vi "RampSlow.vi"() -> ()   [LabVIEW 2016]
uses:
  controls/Enum.ctl
  <vilib>/rvi/errors/niLvFpgaAdjustHostInterfaceError.vi
  <vilib>/rvi/interface/nirviReadWriteControl/nirviReadWriteControl.xnode
  controls/FPGAVIreferenceTypeDef.ctl
  FPGA Bitfiles/qnmController797_usbRIO_controllerFPGAmu-19072018.lvbitx
  Course Project/support/Message Queue/Message Queue.lvlib
  controllerFPGA_multiTarget.vi
  <vilib>/rvi/interface/nirviCloseFPGA/nirviCloseFPGA.xnode
  NiFpgaLv.dll
  <vilib>/rvi/interface/nirviMethod/nirviMethod.xnode
  <vilib>/FPGAPlugInAG/USB-7856R OEM/niLvFpga_AcknowledgeIrq_USB-7856R OEM.vi
  <vilib>/rvi/interface/nirviMethod/StockFPGA_InlinedMethodWaitForSingleIRQ.vi
  <vilib>/FPGAPlugInAG/USB-7856R OEM/niLvFpga_WaitOnIrq_USB-7856R OEM.vi
  <vilib>/FPGAPlugInAG/USB-7856R OEM/niLvFpga_Close_USB-7856R OEM.vi
panel:
  in  "SecureTip":T1 {"Sign" items=[">", "<"]; "Secure tip signal" items=["Vert. Deflection (V)", "Horiz. Deflection (V)", "Input 1", "Input 2"]; "Max-min-Tip" format="%#.2p"}
  in  "Curves 2":i32(listbox)
  in  "Spectroscopy":enum32{"Spectroscopy"}(tab)
  in  "Fwd sweep":bool=TRUE
  in  "Parameters":T2={"Start"=-1e-06, "Distance"=2e-07, "Points"=256.0, "Fwd"=0.0, "Bwd"=0.0, "Pause"=0.0} {"Pause" format="%.0ps"; "Bwd" format="%.0pm/s"; "Distance" format="%#.3pm"; "Start" format="%#.3pm"; "Fwd" format="%.0pm/s"}
  in  "ChannelDisplay2":u16(ring)=1 items=["AI0", "AI1", "AI3", "AI2"]
  in  "ChannelDisplay":u16(ring) items=["AI0", "AI1", "AI3", "AI2"]
  in  "Dec":dbl=1.0 format="%.0p"
  out "ForceCurves 2":cluster{dbl[], dbl[]}[](graph)
  out "ForceCurves":cluster{dbl[], dbl[]}[](graph)
  out "Ramping?":bool
  in  "Bwd sweep":bool=TRUE
  in  "Output":enum16{"Z", "Bias", "..."}(ring)
  in  "Channels":i32[](listbox)=[0, 1, 2, 3]
  in  "Actions":T3={"Play"=FALSE, "Stop"=FALSE, "Loop"=FALSE, "Sweeps"=1.0} {"Sweeps" min=1.0 format="%#.0f"}
  in  "Saving":T4={"#"=0, "Name"="", "Path"=path "C:/ForceCurves", "Autosave"=FALSE, "Save"=FALSE} {"#" format="%03.0f"}
  in  "Curves":T5={"Plot1"={"Apply"=FALSE, "Delete"=FALSE, "Show"=TRUE}, "Plot2"={"Apply"=FALSE, "Delete"=FALSE, "Show"=TRUE}}
  in  "CalculateSlope":bool
  out "1/Slope":dbl format="%#_5pm/V"
  out "B":cluster{"Y":dbl, "X":dbl} {"X" format="%#_2p"; "Y" format="%#_2p"}
  out "A":cluster{"Y":dbl, "X":dbl} {"X" format="%#_2p"; "Y" format="%#_2p"}
  # "Secure tip"
  # "Spectroscopy"
  # "Ramp"
  # "Saving"
  # "Cursors"
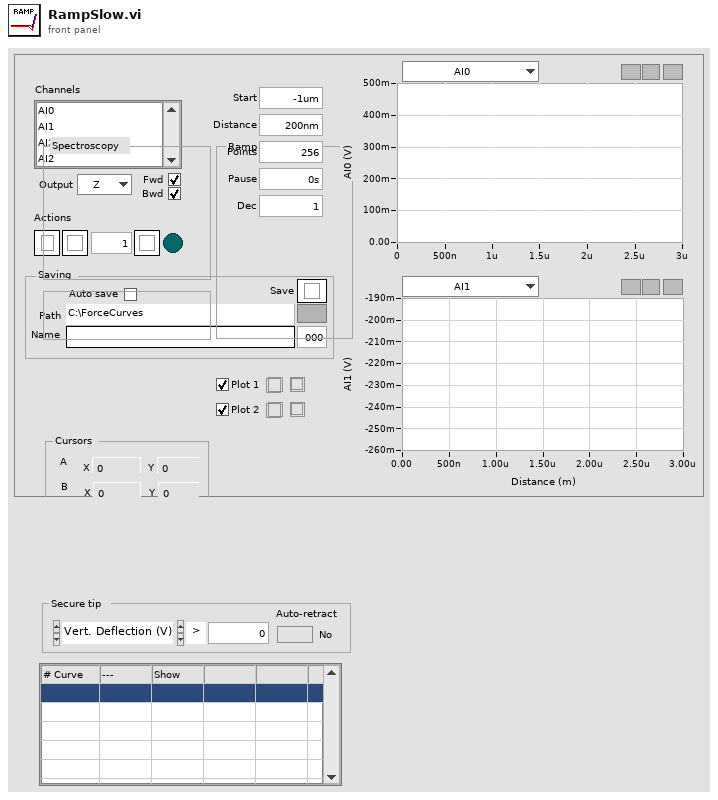
[diagram p1: front panel]
types:
  T1 = cluster{"Max-min-Tip":dbl, "Secure tip signal":u16, "Sign":u16, "Auto-retract":bool}
  T2 = cluster{"Start":dbl, "Distance":dbl, "Points":dbl, "Fwd":dbl, "Bwd":dbl, "Pause":dbl}
  T3 = cluster{"Play":bool, "Stop":bool, "Loop":bool, "Sweeps":dbl}
  T4 = cluster{"#":i64, "Name":string, "Path":path, "Autosave":bool, "Save":bool}
  T5 = cluster{"Plot1":cluster{"Apply":bool, "Delete":bool, "Show":bool}, "Plot2":cluster{"Apply":bool, "Delete":bool, "Show":bool}}
  T6 = typedef "Message Queue.lvlib/All Message Queues.ctl" = cluster{"IU":refnum<queue>}
  T7 = typedef "LVPointDoubleTypeDef.ctl" = cluster{"Cursor X":dbl, "Cursor Y":dbl}
  T8 = typedef "Enum.ctl" = enum16{"Init", "Read", "Write"}
  T9 = enum8{"Enabled", "Disabled", "Disabled and Grayed Out"}
  T10 = enum16{"open", "replace", "create", "open or create", "replace or create", "replace or create with confirmation"}
  T11 = cluster{"calibName":string[], "calibParameters":cluster{"Sensitivity":cluster{"Sens X":dbl, "Sens Y":dbl, "Sens Z":dbl}, "Range":cluster{"Range X":dbl, "Range Y":dbl, "Range Z":dbl}, "HV gain":cluster{"HV gain X":dbl, "HV gain Y":dbl, "HV gain Z":dbl}}[], "calibIndex":i32}
  T12 = cluster{"Sensitivity":cluster{"Sens X":dbl, "Sens Y":dbl, "Sens Z":dbl}, "Range":cluster{"Range X":dbl, "Range Y":dbl, "Range Z":dbl}, "HV gain":cluster{"HV gain X":dbl, "HV gain Y":dbl, "HV gain Z":dbl}}[]
  T13 = cluster{"Sensitivity":cluster{"Sens X":dbl, "Sens Y":dbl, "Sens Z":dbl}, "Range":cluster{"Range X":dbl, "Range Y":dbl, "Range Z":dbl}, "HV gain":cluster{"HV gain X":dbl, "HV gain Y":dbl, "HV gain Z":dbl}}
  T14 = typedef "FPGAVIreferenceTypeDef.ctl" = refnum<k20>
  T15 = cluster{"enableManualMotion":bool, "doMove":bool, "integratorTarget":fxp<+/-,22,2>, "clocks":cluster{"inverseDecimation":fxp<+,22,0>, "decimation":u16, "waveSize":u16, "pixelDecimation":u16}}
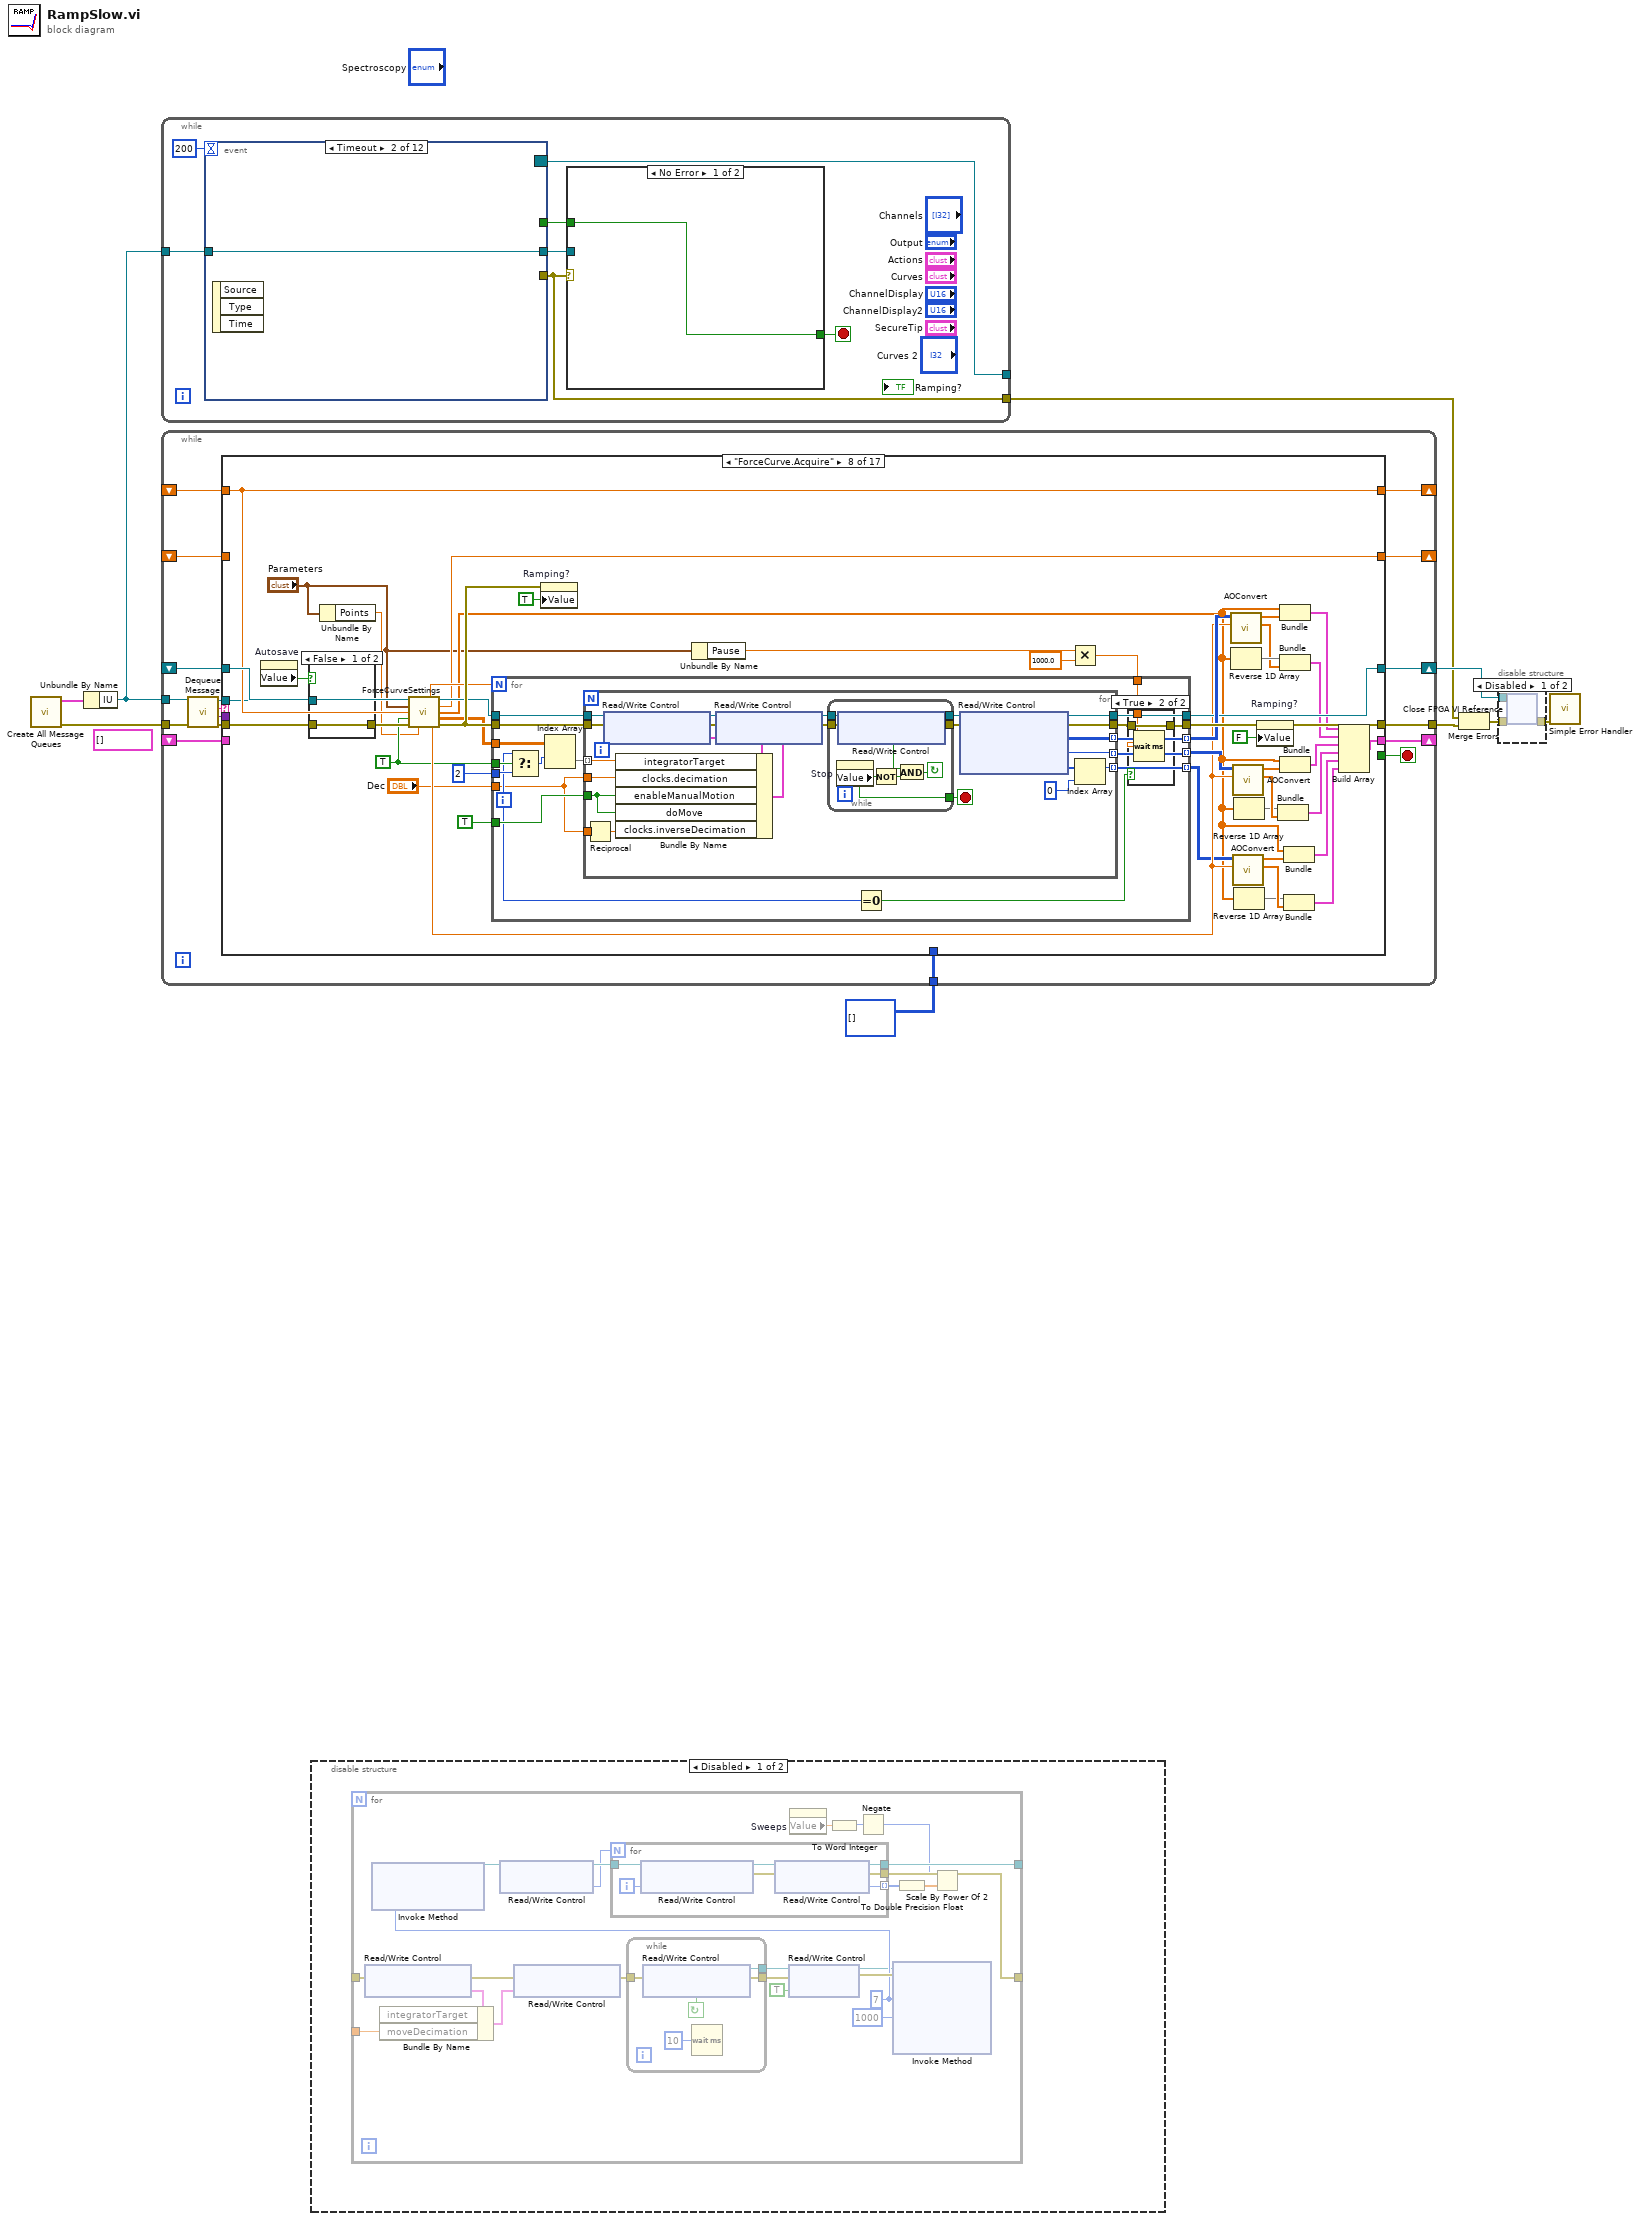
[diagram p0: block diagram]
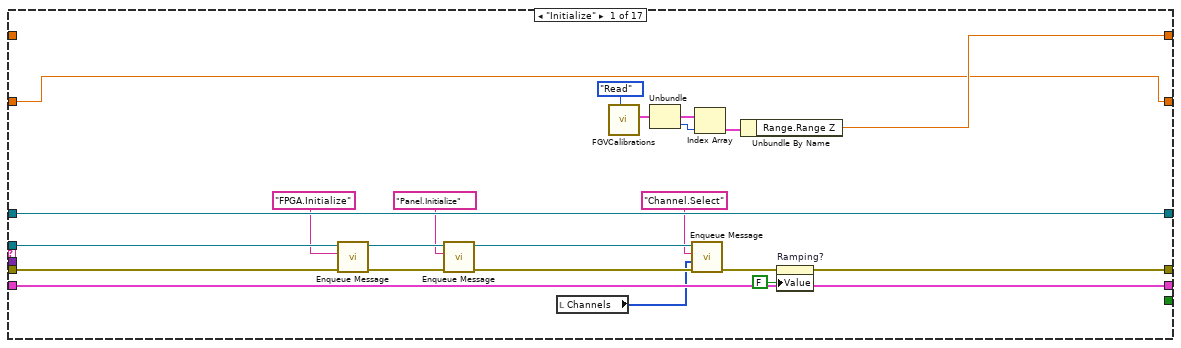
[diagram p4: hidden frame]
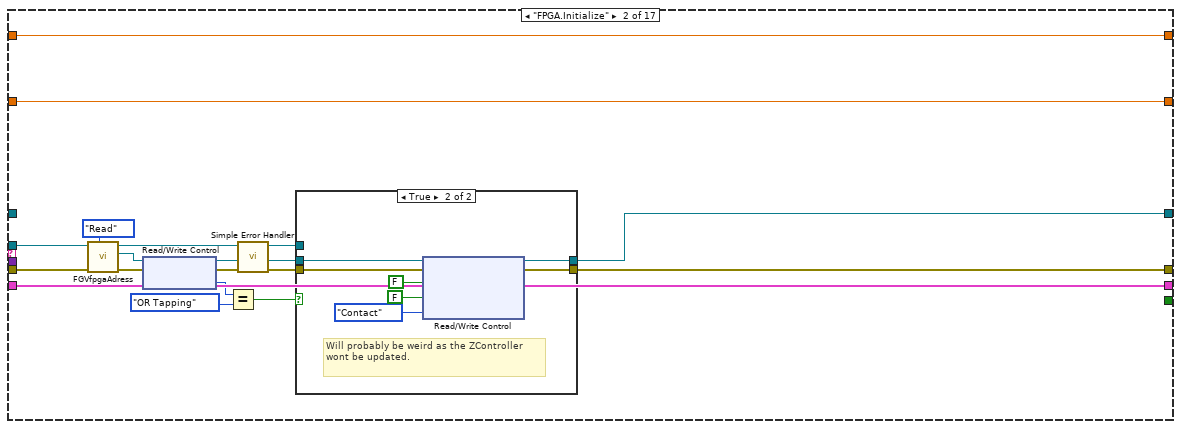
[diagram p5: hidden frame]
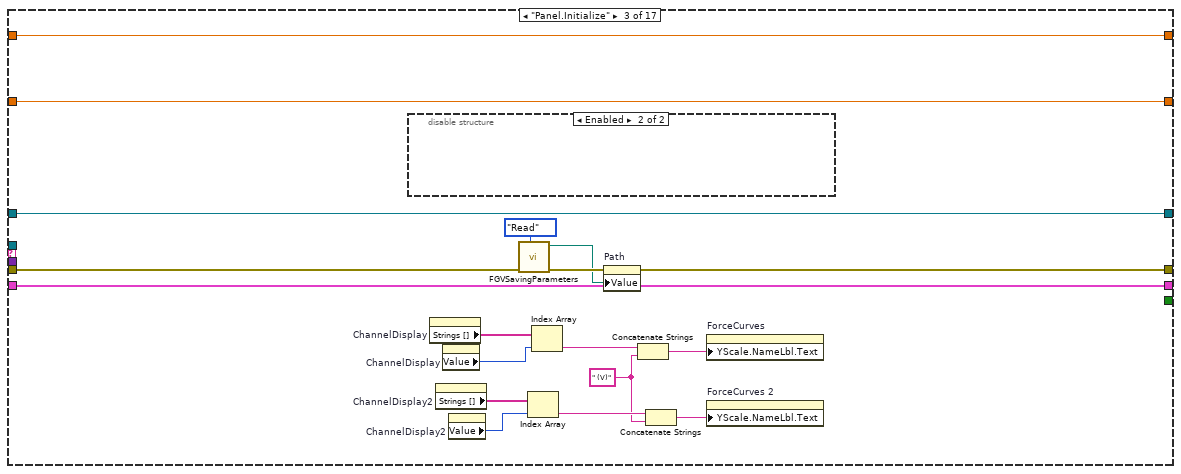
[diagram p7: hidden frame]
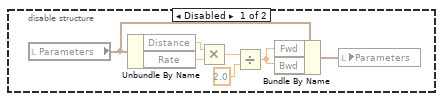
[diagram p8: hidden frame]
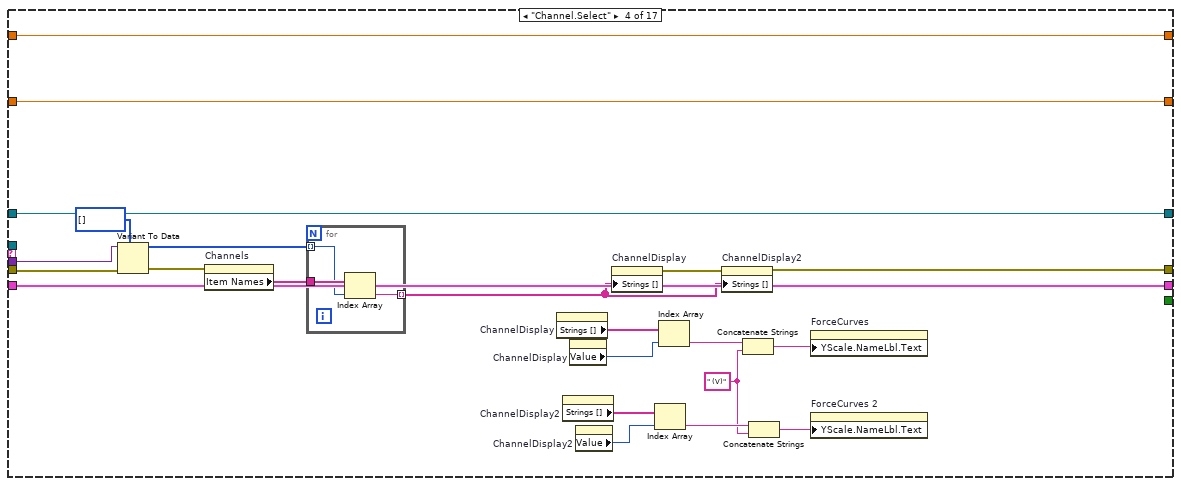
[diagram p9: hidden frame]
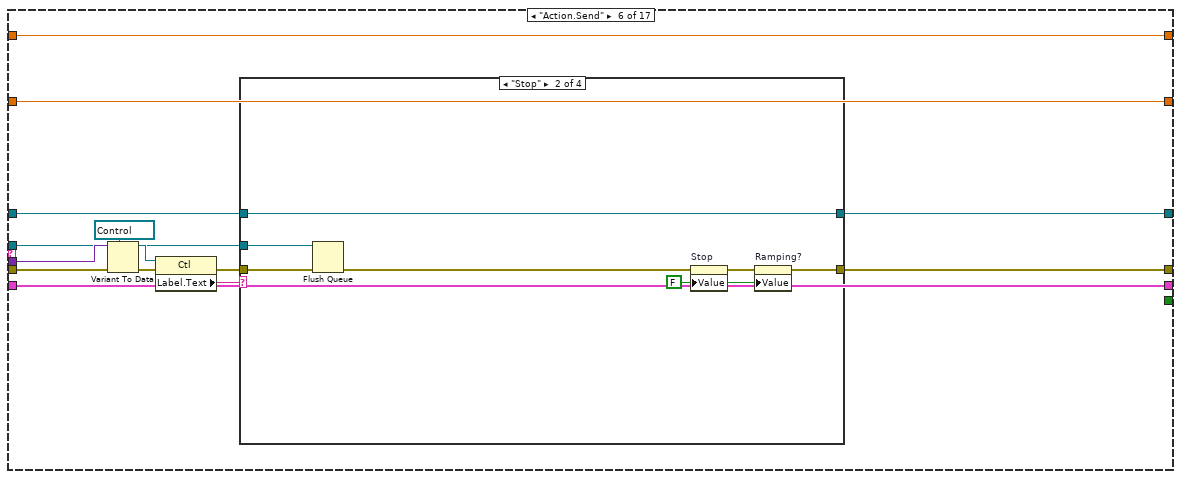
[diagram p11: hidden frame]
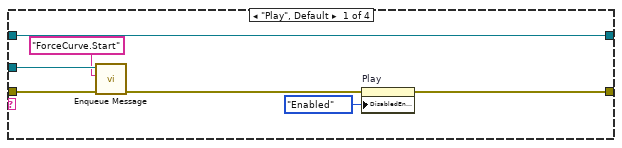
[diagram p12: hidden frame]
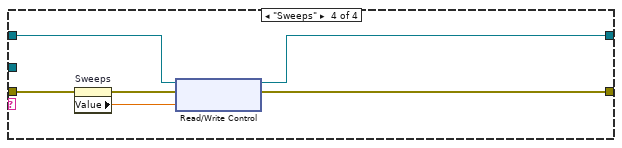
[diagram p14: hidden frame]
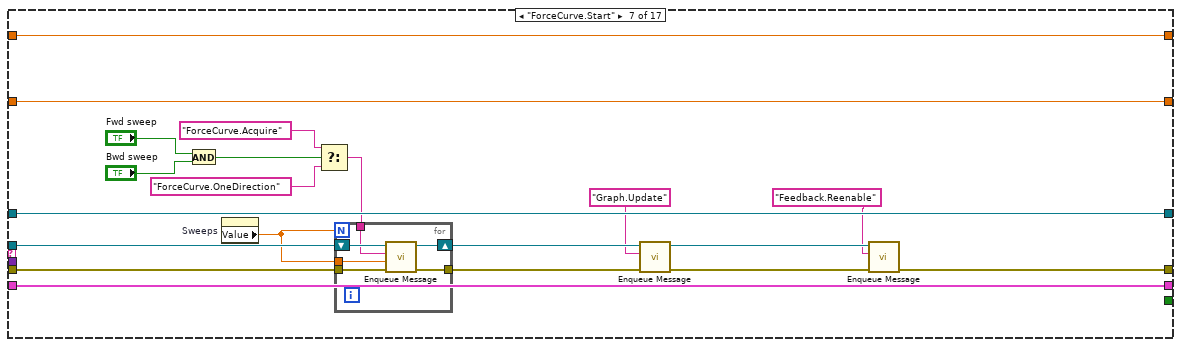
[diagram p15: hidden frame]
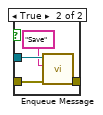
[diagram p16: hidden frame]
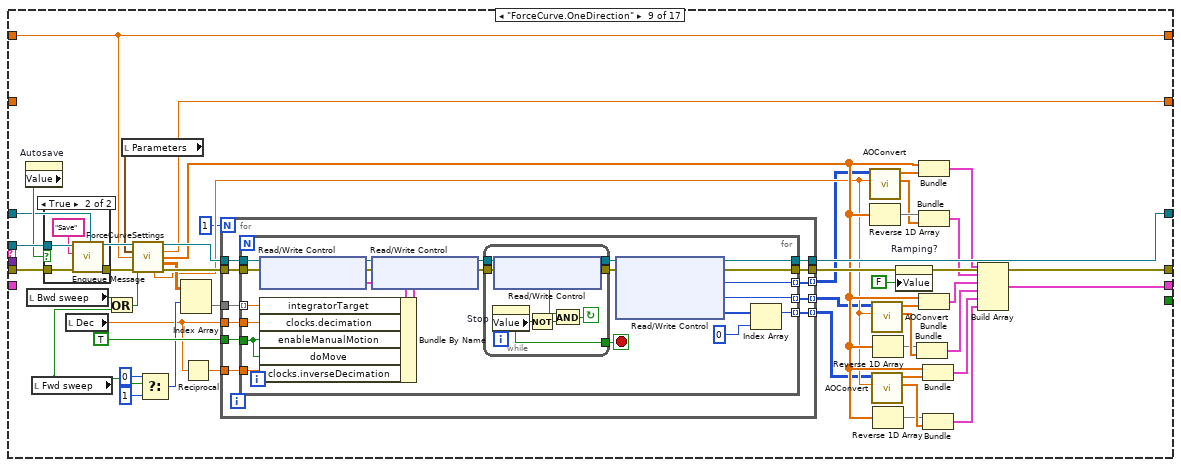
[diagram p18: hidden frame]
diagram:
  (unwired) cluster{dbl[], dbl[]}[] []
  n1 = call "Create All Message Queues.vi"() -> ("ErrorOut"=w4:errorcluster, "MessageQueueOut"=w9:T6)  [unwired: 10 in]
  n2 = Unbundle By Name(w9) -> ("IU"=w3:refnum<queue>)
  n3 = while {
    tunnel: w3 -> [w16]
    tunnel: [w12] -> w2
    tunnel: [w11] -> _
    stop <- w14 stop-if-true
    n4 = event shown="[1] Timeout" {
      selector: _ -> [_ _ _ _ _ _ _ _ _ _ _ _]
      dyn-events: [_ _ _ _ _ _ _ _ _ _ _ _] -> w11
      timeout: 200 -> [_ _ _ _ _ _ _ _ _ _ _ _]
      tunnel: [w27 _ _ _ _ _ _ _ _ _ _ _] -> w15
      tunnel: w16 -> [w22 w28 w34 w37 w42 w46 w50 w55 w59 w68 w72 w77]
      tunnel: [w26 _ w32 _ w39 w43 _ w52 _ _ w69 _] -> w12
      tunnel: [w25 w28 w33 w36 w40 w45 w48 w54 w59 w68 w71 w76] -> w13
      event Panel Close? {
        (unwired) FALSE
        (unwired) TRUE ("Prioritary message")
        w27 = TRUE ("Rejeter ?")
        n5 = event-data() -> ()  [unwired: 1 in, 1 out]
        n6 = call "Enqueue Message.vi"("Prioritary message"=TRUE ("Message prioritaire ? (F)"), "Message"="Exit", "Queue"=w22) -> ("error out"=w26:errorcluster, "Queue dup."=w25:refnum<queue>)  [unwired: 7 in]
        n7 = event-data ("Event Filter Node")("Discard?"=w27) -> ()  [unwired: 1 in, 1 out]
      }
      event Timeout {
        n8 = event-data() -> ()  [unwired: 1 in, 3 out]
      }
      event "Actions.Sweeps", "Actions.Loop": Value Change; "Actions.Play", "Actions.Stop": Mouse Down {
        n9 = event-data() -> ("CtlRef"=w30:refnum<vi>)  [unwired: 1 in]
        n10 = call "Enqueue Message.vi"("Prioritary message"=TRUE, "Data"=w30, "Message"="Action.Send", "Queue"=w34) -> ("error out"=w32:errorcluster, "Queue dup."=w33:refnum<queue>)  [unwired: 6 in]
      }
      event "Parameters.Distance": Value Change {
        n11 = event-data() -> ()  [unwired: 1 in, 6 out]
        n12 = call "Enqueue Message.vi"("Message"="Panel.Initialize", "Queue"=w37) -> ("Queue dup."=w36:refnum<queue>)  [unwired: 8 in, 1 out]
      }
      event "ChannelDisplay", "ChannelDisplay2": Value Change {
        n13 = event-data() -> ("NewVal"=w38:u16)  [unwired: 1 in]
        n14 = call "Enqueue Message.vi"("Data"=w38, "Message"="Graph.Update", "Queue"=w42) -> ("error out"=w39:errorcluster, "Queue dup."=w40:refnum<queue>)  [unwired: 7 in]
      }
      event "Saving.Save": Mouse Down {
        n15 = event-data() -> ()  [unwired: 1 in, 1 out]
        n16 = call "Enqueue Message.vi"("Message"="Save", "Queue"=w46) -> ("error out"=w43:errorcluster, "Queue dup."=w45:refnum<queue>)  [unwired: 8 in]
      }
      event "Saving.Name", "Saving.Path": Value Change {
        n17 = event-data() -> ("CtlRef"=w47:refnum<vi>)  [unwired: 1 in]
        n18 = call "Enqueue Message.vi"("Data"=w47, "Message"="Save.ChangeName", "Queue"=w50) -> ("Queue dup."=w48:refnum<queue>)  [unwired: 7 in, 1 out]
      }
      event "Channels": Value Change {
        n19 = event-data() -> ("NewVal"=w51:i32[])  [unwired: 1 in]
        n20 = call "Enqueue Message.vi"("Data"=w51, "Message"="Channel.Select", "Queue"=w55) -> ("error out"=w52:errorcluster, "Queue dup."=w54:refnum<queue>)  [unwired: 7 in]
      }
      event "ForceCurves": Cursor Move {
        n21 = event-data() -> ("CursIdx"=w56:i32, "CursRef"=w58:refnum<vi>)  [unwired: 1 in]
        n22 = property class="Curs"(reference=w58) -> ("Cursor Position"=w57:T7)  [unwired: 1 in, 2 out]
        n23 = case shown="0, Default" w56 {
          tunnel: w57 -> [w60 w61]
          frame 0, Default {
            "A" <- w60
          }
          frame 1 {
            "B" <- w61
          }
        }
      }
      event "CalculateSlope": Mouse Down {
        n24 = event-data() -> ()  [unwired: 1 in, 1 out]
        n25 = property on="A" class="Clust (strict)"() -> ("Value"=w67:cluster{"Y":dbl, "X":dbl})  [unwired: 2 in, 2 out]
        n26 = property on="B" class="Clust (strict)"() -> ("Value"=w66:cluster{"Y":dbl, "X":dbl})  [unwired: 2 in, 2 out]
        n27 = Subtract(x=w67, y=w66) -> (x-y=w65:cluster{"Y":dbl, "X":dbl})
        n28 = Unbundle By Name(w65) -> ("Y"=w64:dbl, "X"=w63:dbl)
        n29 = Divide(x=w64, y=w63) -> (x/y=→"1/Slope":dbl)
      }
      event "ForceCurves", "ForceCurves 2": Value Change {
        n30 = event-data() -> ()  [unwired: 1 in, 1 out]
        n31 = call "Enqueue Message.vi"("Message"="Graph.Update", "Queue"=w72) -> ("error out"=w69:errorcluster, "Queue dup."=w71:refnum<queue>)  [unwired: 8 in]
      }
      event "Curves.Plot1.Apply", "Curves.Plot2.Apply": Mouse Down {
        n32 = event-data() -> ("CtlRef"=w74:refnum<vi>)  [unwired: 1 in]
        n33 = To Variant(anything=w74) -> (Variant=w73:variant)
        n34 = call "Enqueue Message.vi"("Data"=w73, "Message"="SaveToImage", "Queue"=w77) -> ("Queue dup."=w76:refnum<queue>)  [unwired: 7 in, 1 out]
      }
    }
    n35 = case shown="No Error" w12 {
      tunnel: [w17 TRUE ("Rejeter ?")] -> w14
      tunnel: w15 -> [w17 _]
      tunnel: w13 -> [_ w20]
      frame No Error {
      }
      frame Error {
        n36 = call "Enqueue Message.vi"("Prioritary message"=TRUE ("Message prioritaire ? (F)"), "Message"="Exit", "Queue"=w20) -> ()  [unwired: 7 in, 2 out]
      }
    }
  }
  n37 = while {
    shift-right: [w90] -> w5
    shift-left: _ -> [w89]
    tunnel: [w88] -> w6
    tunnel: w4 -> [w86]
    tunnel: w3 -> [w85]
    shift-right: [w84] -> _
    shift-left: _ -> [w83]
    shift-right: [w81] -> _
    shift-left: _ -> [w82]
    shift-right: [w80] -> _
    shift-left: _ -> [w79]
    tunnel: i16[][] [] -> [w78]
    stop <- w94 stop-if-true
    n38 = call "Dequeue Message.vi"("entrée d'erreur (pas d'erreur)"=w86, "File d'attente de messages"=w85) -> ("sortie d'erreur"=w93:errorcluster, "Données de message"=w92:variant, "Message"=w87:string, "File d'attente de message dup."=w91:refnum<queue>)  [unwired: 6 in]
    n39 = case shown="\"ForceCurve.Acquire\"" w87 {
      selector: w87 -> [_ _ _ _ _ _ _ _ _ _ _ _ _ _ _ _ w689]
      tunnel: w91 -> [w113 w129 _ _ _ w201 w251 w267 w403 _ _ _ _ _ _ w681 _]
      tunnel: w93 -> [w114 w131 w149 w182 w196 w210 w246 w269 w401 w459 w486 w497 w574 w643 w668 w678 _]
      tunnel: [w100 w118 w147 w183 w196 w202 w240 w299 w408 w459 w486 w500 w547 w642 w667 w677 w687] -> w88
      tunnel: [_ _ _ _ _ _ _ _ _ _ _ _ _ _ _ TRUE _] -> w94
      tunnel: w92 -> [_ _ _ w180 _ w209 _ _ _ _ _ _ _ w641 _ _ _]
      tunnel: [w115 w119 w158 w188 w195 w198 w250 w298 w407 w458 w485 w499 w573 w646 w672 w676 w685] -> w90
      tunnel: w89 -> [w115 _ w158 w188 w195 w204 w250 w300 w399 w458 w485 w498 w573 w646 w672 w676 w685]
      tunnel: [w111 w132 w157 w187 w194 w200 w249 w296 w365 w457 w475 w511 w518 w647 w671 w675 w684] -> w84
      tunnel: w83 -> [w111 w132 w157 w187 w194 w200 w249 _ _ w457 w475 w511 w518 w647 w671 w675 w684]
      tunnel: w82 -> [_ w120 w156 w186 w193 w199 w248 w286 w397 w456 w484 w510 w572 w645 w670 w674 w683]
      tunnel: [w105 w120 w156 w186 w193 w199 w248 w286 w397 w456 w484 w510 w572 w645 w670 w674 w683] -> w81
      tunnel: [w99 w117 w151 w185 w192 w197 w243 w283 w393 w455 w476 w489 w554 w644 w669 w673 w682] -> w80
      tunnel: w79 -> [w99 w117 w151 w185 w192 w197 w243 _ _ w455 w476 w489 w554 w644 w669 w673 w682]
      tunnel: w78 -> [_ _ _ _ _ _ _ _ _ _ _ _ _ _ _ _ _]
      frame "Initialize" {
        n40 = call "Enqueue Message.vi"("error in"=w114, "Message"="FPGA.Initialize", "Queue"=w113) -> ("error out"=w103:errorcluster, "Queue dup."=w102:refnum<queue>)  [unwired: 7 in]
        n41 = call "Enqueue Message.vi"("error in"=w103, "Message"="Panel.Initialize", "Queue"=w102) -> ("error out"=w97:errorcluster, "Queue dup."=w116:refnum<queue>)  [unwired: 7 in]
        n42 = local read "Channels"() -> (w95:i32[])
        n43 = call "FGVCalibrations.vi"("Enum"=Enum."Read") -> ("calibOut"=w109:T11)  [unwired: 9 in, 1 out]
        n44 = Unbundle(w109) -> ("calibParameters"=w107:T12, "calibIndex"=w106:i32)  [unwired: 1 out]
        n45 = call "Enqueue Message.vi"("error in"=w97, "Data"=w95, "Message"="Channel.Select", "Queue"=w116) -> ("error out"=w96:errorcluster)  [unwired: 6 in, 1 out]
        n46 = Index Array(array=w107, index=w106) -> (element=w110:T13)
        n47 = Unbundle By Name(w110) -> ("Range.Range Z"=w105:dbl)
        n48 = property on="Ramping?" class="Bool (strict)"(error in=w96, "Value"=FALSE ("Ramping?")) -> (error out=w100:errorcluster)  [unwired: 1 in, 1 out]
      }
      frame "FPGA.Initialize" {
        n49 = call "FGVfpgaAdress.vi"("Enum"=Enum."Read", "error in"=w131) -> ("error out"=w122:errorcluster, "FPGA VI Reference Out"=w128:T14)  [unwired: 5 in, 3 out]
        n50 = xnode "Read/Write Control"("FPGA VI Reference In"=w128, "error in"=w122) -> ("FPGA VI Reference Out"=w127:T14, "error out"=w123:errorcluster, "fb.i.source"=w126:u8)
        n51 = Equal?(x=w126, y=enum16{"Contact", "OR Tapping", "Aux"}."OR Tapping" ("Mode")) -> (x = y?=w124:bool)
        n52 = call <vilib>:"Simple Error Handler.vi"("error in (no error)"=w123) -> ("error out"=w121:errorcluster)  [unwired: 4 in, 4 out]
        n53 = case shown="True" w124 {
          tunnel: [w133 w138] -> w118
          tunnel: [w134 w140] -> w119
          tunnel: w127 -> [w134 w141]
          tunnel: w129 -> [_ _]
          tunnel: w121 -> [w133 w137]
          frame False {
          }
          frame True {
            # "Will probably be weird as the ZController wont be updated."
            n54 = xnode "Read/Write Control"("FPGA VI Reference In"=w141, "error in"=w137, "fb.p.enable"=FALSE, "aio.o.disableExc"=FALSE, "fb.i.source"=enum16{"Contact", "OR Tapping", "Aux"}."Contact" ("Mode")) -> ("FPGA VI Reference Out"=w140:T14, "error out"=w138:errorcluster)
          }
        }
      }
      frame "Panel.Initialize" {
        w142 = " (V)" ("Y Scale.Unit Label.Text")
        n55 = disable-structure shown="Enabled" {
          frame Disabled {
            n56 = local read "Parameters"() -> (w164:T2)
            n57 = Unbundle By Name(w164) -> ("Distance"=w165:dbl, "Rate"=w166:dbl)
            n58 = Multiply(x=w165, y=w166) -> (x*y=w162:dbl)
            n59 = Divide(x=w162, y=2.0) -> (x/y=w161:dbl)
            n60 = Bundle By Name(cluster=w164, "Fwd"=w161, "Bwd"=w161) -> (w163:T2)
            n61 = local write "Parameters"(w163) -> ()
          }
          frame Enabled {
          }
        }
        n62 = property on="ChannelDisplay" class="Ring (strict)"() -> ("Strings []"=w155:string[])  [unwired: 2 in, 2 out]
        n63 = property on="ChannelDisplay2" class="Ring (strict)"() -> ("Strings []"=w154:string[])  [unwired: 2 in, 2 out]
        n64 = property on="ChannelDisplay" class="Ring (strict)"() -> ("Value"=w152:u16)  [unwired: 2 in, 2 out]
        n65 = property on="ChannelDisplay2" class="Ring (strict)"() -> ("Value"=w153:u16)  [unwired: 2 in, 2 out]
        n66 = call "FGVSavingParameters.vi"("Enum"=Enum."Read", "error in"=w149) -> ("error out"=w159:errorcluster, "pathOut"=w148:path)  [unwired: 6 in, 2 out]
        n67 = Index Array(array=w154, index=w153) -> (element=w145:string)
        n68 = Index Array(array=w155, index=w152) -> (element=w146:string)
        n69 = property on="Path" class="Path"(error in=w159, "Value"=w148) -> (error out=w147:errorcluster)  [unwired: 1 in, 1 out]
        n70 = Concatenate Strings(w146, w142) -> (w143:string)
        n71 = Concatenate Strings(w145, w142) -> (w144:string)
        n72 = property on="ForceCurves" class="XYGraph (strict)"("YScale.NameLbl.Text"=w143) -> ()  [unwired: 2 in, 2 out]
        n73 = property on="ForceCurves 2" class="XYGraph (strict)"("YScale.NameLbl.Text"=w144) -> ()  [unwired: 2 in, 2 out]
      }
      frame "Channel.Select" {
        w167 = " (V)" ("Y Scale.Unit Label.Text")
        n74 = Variant To Data(error in=w182, type=i32[] [] ("NewVal"), Variant=w180) -> (data=w177:i32[], error out=w179:errorcluster)
        n75 = property on="Channels" class="LstBox (strict)"(error in=w179) -> ("Item Names"=w178:string[])  [unwired: 1 in, 2 out]
        n76 = for {
          tunnel: w178 -> [w191]
          tunnel: w177 -> [w190] mode=indexing
          tunnel: [w189] -> w176 mode=indexing
          n77 = Index Array(array=w191, index=w190) -> (element=w189:string)
        }
        n78 = property on="ChannelDisplay" class="Ring (strict)"() -> ("Strings []"=w175:string[])  [unwired: 2 in, 2 out]
        n79 = property on="ChannelDisplay2" class="Ring (strict)"() -> ("Strings []"=w174:string[])  [unwired: 2 in, 2 out]
        n80 = property on="ChannelDisplay" class="Ring (strict)"() -> ("Value"=w172:u16)  [unwired: 2 in, 2 out]
        n81 = property on="ChannelDisplay2" class="Ring (strict)"() -> ("Value"=w173:u16)  [unwired: 2 in, 2 out]
        n82 = property on="ChannelDisplay" class="Ring (strict)"("Strings []"=w176) -> (error out=w184:errorcluster)  [unwired: 2 in, 1 out]
        n83 = Index Array(array=w174, index=w173) -> (element=w171:string)
        n84 = Index Array(array=w175, index=w172) -> (element=w170:string)
        n85 = property on="ChannelDisplay2" class="Ring (strict)"(error in=w184, "Strings []"=w176) -> (error out=w183:errorcluster)  [unwired: 1 in, 1 out]
        n86 = Concatenate Strings(w170, w167) -> (w169:string)
        n87 = Concatenate Strings(w171, w167) -> (w168:string)
        n88 = property on="ForceCurves" class="XYGraph (strict)"("YScale.NameLbl.Text"=w169) -> ()  [unwired: 2 in, 2 out]
        n89 = property on="ForceCurves 2" class="XYGraph (strict)"("YScale.NameLbl.Text"=w168) -> ()  [unwired: 2 in, 2 out]
      }
      frame "Channel.Display" {
      }
      frame "Action.Send" {
        n90 = Variant To Data(error in=w210, type=refnum<vi> refnum ("CtlRef"), Variant=w209) -> (data=w207:refnum<vi>, error out=w206:errorcluster)
        n91 = property class="Ctl"(reference=w207, error in=w206) -> (error out=w203:errorcluster, "Label.Text"=w205:string)  [unwired: 1 out]
        n92 = case shown="\"Stop\"" w205 {
          tunnel: w204 -> [w214 w218 w226 w232]
          tunnel: w203 -> [w215 w220 w225 w230]
          tunnel: [w212 w223 w225 w228] -> w202
          tunnel: [w214 w218 w226 w227] -> w198
          tunnel: w201 -> [w217 w221 _ _]
          frame "Play", Default {
            n93 = call "Enqueue Message.vi"("error in"=w215, "Message"="ForceCurve.Start", "Queue"=w217) -> ("error out"=w213:errorcluster)  [unwired: 7 in, 1 out]
            n94 = property on="Play" class="Bool (strict)"(error in=w213, "DisabledEnum"=T9."Enabled" ("Disabled")) -> (error out=w212:errorcluster)  [unwired: 1 in, 1 out]
          }
          frame "Stop" {
            w222 = FALSE ("Value")
            n95 = Flush Queue(queue=w221, error in (no error)=w220) -> (error out=w219:errorcluster)  [unwired: 2 out]
            n96 = property on="Stop" class="Bool (strict)"(error in=w219, "Value"=w222) -> (error out=w224:errorcluster)  [unwired: 1 in, 1 out]
            n97 = property on="Ramping?" class="Bool (strict)"(error in=w224, "Value"=w222) -> (error out=w223:errorcluster)  [unwired: 1 in, 1 out]
          }
          frame "Continuous" {
          }
          frame "Sweeps" {
            n98 = property on="Sweeps" class="DigNum (strict)"(error in=w230) -> (error out=w229:errorcluster, "Value"=w231:dbl)  [unwired: 1 in, 1 out]
            n99 = xnode "Read/Write Control"("FPGA VI Reference In"=w232, "error in"=w229, "lwr.p.avgCnt"=w231) -> ("FPGA VI Reference Out"=w227:T14, "error out"=w228:errorcluster)
          }
        }
      }
      frame "ForceCurve.Start" {
        n100 = And(x="Fwd sweep", y="Bwd sweep") -> (x .and. y?=w233:bool)
        n101 = property on="Sweeps" class="DigNum (strict)"() -> ("Value"=w245:dbl)  [unwired: 2 in, 2 out]
        n102 = Select(t="ForceCurve.Acquire" ("Message"), s=w233, f="ForceCurve.OneDirection" ("Message")) -> (s? t:f=w236:string)
        n103 = for {
          N: w245 -> [_]
          shift-right: [w257] -> w252
          shift-left: w251 -> [w258]
          tunnel: w246 -> [w255]
          tunnel: [w256] -> w244
          tunnel: w245 -> [w254]
          tunnel: w236 -> [w253]
          n104 = call "Enqueue Message.vi"("error in"=w255, "Data"=w254, "Message"=w253, "Queue"=w258) -> ("error out"=w256:errorcluster, "Queue dup."=w257:refnum<queue>)  [unwired: 6 in]
        }
        n105 = call "Enqueue Message.vi"("error in"=w244, "Message"="Graph.Update", "Queue"=w252) -> ("error out"=w241:errorcluster, "Queue dup."=w242:refnum<queue>)  [unwired: 7 in]
        n106 = call "Enqueue Message.vi"("error in"=w241, "Message"="Feedback.Reenable", "Queue"=w242) -> ("error out"=w240:errorcluster)  [unwired: 7 in, 1 out]
      }
      frame "ForceCurve.Acquire" {
        w261 = TRUE ("Bwd sweep")
        n107 = property on="Autosave" class="Bool (strict)"() -> ("Value"=w266:bool)  [unwired: 2 in, 2 out]
        n108 = case shown="False" w266 {
          tunnel: w269 -> [w305 w309]
          tunnel: [w305 w308] -> w268
          tunnel: w267 -> [_ w307]
          frame False {
          }
          frame True {
            n109 = call "Enqueue Message.vi"("error in"=w309, "Message"="Save", "Queue"=w307) -> ("error out"=w308:errorcluster)  [unwired: 7 in, 1 out]
          }
        }
        n110 = Unbundle By Name("Parameters") -> ("Points"=w259:dbl)
        n111 = call "ForceCurveSettings.vi"("FPGA ref in"=w300, "Parameters"="Parameters", "Range Z"=w286, "Bwd sweep"=w261, "error in"=w268, "Points"=w259) -> ("BwdSweep(T=2, F=1)"=w302:dbl, "FPGA ref out"=w297:T14, "Zheight"=w283:dbl, "PointsArray"=w271:dbl[], "RampDistancePoints"=w282:dbl[][], "Voltage Range"=w275:dbl, "error out"=w303:errorcluster)  [unwired: 3 in]
        n112 = property on="Ramping?" class="Bool (strict)"(error in=w303, "Value"=TRUE ("Ramping?")) -> ()  [unwired: 1 in, 2 out]
        n113 = Unbundle By Name("Parameters") -> ("Pause"=w264:dbl)
        n114 = Multiply(x=w264, y=1000.0) -> (x*y=w263:dbl)
        n115 = for {
          N: w302 -> [_]
          tunnel: [w324] -> w301 mode=indexing
          tunnel: [w323] -> w291 mode=indexing
          tunnel: TRUE ("enableManualMotion") -> [w322]
          tunnel: w303 -> [w327]
          tunnel: [w314] -> w304
          tunnel: w297 -> [w325]
          tunnel: [w326] -> w298
          tunnel: "Dec" -> [w310]
          tunnel: [w321] -> w274 mode=indexing
          tunnel: w282 -> [w320]
          tunnel: w261 -> [w317]
          tunnel: 2 ("f") -> [w316]
          tunnel: w263 -> [w313]
          i -> [w311]
          n116 = Select(t=w311, s=w317, f=w316) -> (s? t:f=w318:i32)
          n117 = Index Array(array=w320, index (row)=w318) -> (element=w319:dbl[])  [unwired: 1 in]
          n118 = for {
            tunnel: [w337] -> w324 mode=indexing
            tunnel: [w347] -> w323 mode=indexing
            tunnel: [w346] -> w315
            tunnel: [w345] -> w326
            tunnel: w327 -> [w344]
            tunnel: w325 -> [w341]
            tunnel: w322 -> [w340]
            tunnel: w310 -> [w333]
            tunnel: [w335] -> w321 mode=indexing
            tunnel: w319 -> [w336] mode=indexing
            tunnel: w310 -> [w331]
            stop <- w339 stop-if-true
            n119 = Reciprocal(x=w331) -> (1/x=w332:dbl)
            n120 = xnode "Read/Write Control"("FPGA VI Reference In"=w341, "error in"=w344) -> ("FPGA VI Reference Out"=w343:T14, "error out"=w353:errorcluster, "fb.mot.p.params"=w352:T15)
            n121 = Bundle By Name(cluster=w352, "integratorTarget"=w336, "clocks.decimation"=w333, "enableManualMotion"=w340, "doMove"=w340, "clocks.inverseDecimation"=w332) -> (w351:T15)
            n122 = xnode "Read/Write Control"("FPGA VI Reference In"=w343, "error in"=w353, "fb.mot.p.params"=w351) -> ("FPGA VI Reference Out"=w342:T14, "error out"=w350:errorcluster)
            n123 = while {
              tunnel: w350 -> [w361]
              tunnel: [w360] -> w349
              tunnel: [w359] -> w348
              tunnel: w342 -> [w358]
              tunnel: [w354] -> w339
              stop <- w357 continue-if-true
              n124 = property on="Stop" class="Bool (strict)"() -> ("Value"=w354:bool)  [unwired: 2 in, 2 out]
              n125 = xnode "Read/Write Control"("FPGA VI Reference In"=w358, "error in"=w361) -> ("FPGA VI Reference Out"=w360:T14, "error out"=w359:errorcluster, "fb.mot.s.running"=w356:bool)
              n126 = Not(x=w354) -> (.not. x?=w355:bool)
              n127 = And(x=w356, y=w355) -> (x .and. y?=w357:bool)
            }
            n128 = xnode "Read/Write Control"("FPGA VI Reference In"=w349, "error in"=w348) -> ("FPGA VI Reference Out"=w345:T14, "error out"=w346:errorcluster, "aio.s.slowVertical"=w337:i16, "aio.s.slowHoriz"=w347:i16, "aio.o.inputs"=w338:i16[])
            n129 = Index Array(array=w338, index=0) -> (element=w335:i16)
          }
          n130 = Equal To 0?(x=w311) -> (x = 0?=w312:bool)
          n131 = case shown="True" w312 {
            tunnel: w315 -> [w328 w330]
            tunnel: [w328 w330] -> w314
            tunnel: w313 -> [_ w329]
            frame False {
            }
            frame True {
              n132 = Wait (ms)(milliseconds to wait=w329) -> ()  [unwired: 1 out]
            }
          }
        }
        n133 = call "AOConvert.vi"("Voltage Range"=w275, "Signal"=w301) -> ("Retract"=w284:dbl[], "Approach"=w285:dbl[])  [unwired: 8 in]
        n134 = Reverse 1D Array(array=w271) -> (reversed array=w289:dbl[])
        n135 = call "AOConvert.vi"("Voltage Range"=w275, "Signal"=w291) -> ("Retract"=w288:dbl[], "Approach"=w290:dbl[])  [unwired: 8 in]
        n136 = call "AOConvert.vi"("Voltage Range"=w275, "Signal"=w274) -> ("Retract"=w277:dbl[], "Approach"=w278:dbl[])  [unwired: 8 in]
        n137 = Reverse 1D Array(array=w271) -> (reversed array=w287:dbl[])
        n138 = Reverse 1D Array(array=w271) -> (reversed array=w276:dbl[])
        n139 = property on="Ramping?" class="Bool (strict)"(error in=w304, "Value"=FALSE ("Ramping?")) -> (error out=w299:errorcluster)  [unwired: 1 in, 1 out]
        n140 = Bundle(w287, "Retract"=w288) -> (w279:cluster{dbl[], "Retract":dbl[]})  [unwired: 1 in]
        n141 = Bundle("PointsArray"=w271, "Approach"=w285) -> (w293:cluster{"PointsArray":dbl[], "Approach":dbl[]})  [unwired: 1 in]
        n142 = Bundle(w289, "Retract"=w284) -> (w292:cluster{dbl[], "Retract":dbl[]})  [unwired: 1 in]
        n143 = Bundle("PointsArray"=w271, "Approach"=w290) -> (w280:cluster{"PointsArray":dbl[], "Approach":dbl[]})  [unwired: 1 in]
        n144 = Bundle("PointsArray"=w271, "Approach"=w278) -> (w273:cluster{"PointsArray":dbl[], "Approach":dbl[]})  [unwired: 1 in]
        n145 = Bundle(w276, "Retract"=w277) -> (w272:cluster{dbl[], "Retract":dbl[]})  [unwired: 1 in]
        n146 = Build Array(w293, w292, w280, w279, w273, w272) -> (w296:cluster{"PointsArray":dbl[], "Retract":dbl[]}[])
      }
      frame "ForceCurve.OneDirection" {
        n147 = property on="Autosave" class="Bool (strict)"() -> ("Value"=w402:bool)  [unwired: 2 in, 2 out]
        n148 = local read "Bwd sweep"() -> (w392:bool)
        n149 = local read "Fwd sweep"() -> (w390:bool)
        n150 = case shown="True" w402 {
          tunnel: w401 -> [w450 w454]
          tunnel: [w450 w453] -> w404
          tunnel: w403 -> [_ w452]
          frame False {
          }
          frame True {
            n151 = call "Enqueue Message.vi"("error in"=w454, "Message"="Save", "Queue"=w452) -> ("error out"=w453:errorcluster)  [unwired: 7 in, 1 out]
          }
        }
        n152 = local read "Dec"() -> (w362:dbl)
        n153 = Or(x=w392, y=w390) -> (x .or. y?=w391:bool)
        n154 = local read "Parameters"() -> (w395:T2)
        n155 = call "ForceCurveSettings.vi"("FPGA ref in"=w399, "Parameters"=w395, "Range Z"=w397, "Bwd sweep"=w391, "error in"=w404) -> ("FPGA ref out"=w398:T14, "Zheight"=w393:dbl, "PointsArray"=w373:dbl[], "RampDistancePoints"=w396:dbl[][], "Voltage Range"=w372:dbl, "error out"=w405:errorcluster)  [unwired: 4 in, 1 out]
        n156 = Select(t=0, s=w390, f=1) -> (s? t:f=w387:i32)
        n157 = Index Array(array=w396, index (row)=w387) -> (element=w394:dbl[])  [unwired: 1 in]
        n158 = Reciprocal(x=w362) -> (1/x=w363:dbl)
        n159 = for {
          N: 1 -> [_]
          tunnel: w405 -> [w419]
          tunnel: TRUE ("enableManualMotion") -> [w418]
          tunnel: w362 -> [w417]
          tunnel: w398 -> [w416]
          tunnel: w394 -> [w415]
          tunnel: [w414] -> w371 mode=indexing
          tunnel: [w413] -> w370 mode=indexing
          tunnel: [w412] -> w406
          tunnel: [w411] -> w369 mode=indexing
          tunnel: [w410] -> w407
          tunnel: w363 -> [w409]
          n160 = for {
            tunnel: [w425] -> w414 mode=indexing
            tunnel: [w435] -> w413 mode=indexing
            tunnel: [w434] -> w412
            tunnel: [w433] -> w410
            tunnel: w419 -> [w432]
            tunnel: w416 -> [w429]
            tunnel: w418 -> [w428]
            tunnel: w417 -> [w426]
            tunnel: [w422] -> w411 mode=indexing
            tunnel: w415 -> [w424] mode=indexing
            tunnel: w409 -> [w420]
            stop <- w427 stop-if-true
            n161 = xnode "Read/Write Control"("FPGA VI Reference In"=w429, "error in"=w432) -> ("FPGA VI Reference Out"=w431:T14, "error out"=w441:errorcluster, "fb.mot.p.params"=w440:T15)
            n162 = Bundle By Name(cluster=w440, "integratorTarget"=w424, "clocks.decimation"=w426, "enableManualMotion"=w428, "doMove"=w428, "clocks.inverseDecimation"=w420) -> (w439:T15)
            n163 = xnode "Read/Write Control"("FPGA VI Reference In"=w431, "error in"=w441, "fb.mot.p.params"=w439) -> ("FPGA VI Reference Out"=w430:T14, "error out"=w438:errorcluster)
            n164 = while {
              tunnel: w438 -> [w449]
              tunnel: [w448] -> w437
              tunnel: [w447] -> w436
              tunnel: w430 -> [w446]
              tunnel: [w442] -> w427
              stop <- w445 continue-if-true
              n165 = property on="Stop" class="Bool (strict)"() -> ("Value"=w442:bool)  [unwired: 2 in, 2 out]
              n166 = xnode "Read/Write Control"("FPGA VI Reference In"=w446, "error in"=w449) -> ("FPGA VI Reference Out"=w448:T14, "error out"=w447:errorcluster, "fb.mot.s.running"=w444:bool)
              n167 = Not(x=w442) -> (.not. x?=w443:bool)
              n168 = And(x=w444, y=w443) -> (x .and. y?=w445:bool)
            }
            n169 = xnode "Read/Write Control"("FPGA VI Reference In"=w437, "error in"=w436) -> ("FPGA VI Reference Out"=w433:T14, "error out"=w434:errorcluster, "aio.s.slowVertical"=w425:i16, "aio.s.slowHoriz"=w435:i16, "aio.o.inputs"=w423:i16[])
            n170 = Index Array(array=w423, index=0) -> (element=w422:i16)
          }
        }
        n171 = call "AOConvert.vi"("Voltage Range"=w372, "Signal"=w371) -> ("Retract"=w379:dbl[], "Approach"=w380:dbl[])  [unwired: 8 in]
        n172 = Reverse 1D Array(array=w373) -> (reversed array=w383:dbl[])
        n173 = call "AOConvert.vi"("Voltage Range"=w372, "Signal"=w370) -> ("Retract"=w382:dbl[], "Approach"=w384:dbl[])  [unwired: 8 in]
        n174 = call "AOConvert.vi"("Voltage Range"=w372, "Signal"=w369) -> ("Retract"=w376:dbl[], "Approach"=w377:dbl[])  [unwired: 8 in]
        n175 = Reverse 1D Array(array=w373) -> (reversed array=w381:dbl[])
        n176 = Reverse 1D Array(array=w373) -> (reversed array=w375:dbl[])
        n177 = property on="Ramping?" class="Bool (strict)"(error in=w406, "Value"=FALSE ("Ramping?")) -> (error out=w408:errorcluster)  [unwired: 1 in, 1 out]
        n178 = Bundle(w381, "Retract"=w382) -> (w378:cluster{dbl[], "Retract":dbl[]})  [unwired: 1 in]
        n179 = Bundle("PointsArray"=w373, "Approach"=w380) -> (w366:cluster{"PointsArray":dbl[], "Approach":dbl[]})  [unwired: 1 in]
        n180 = Bundle(w383, "Retract"=w379) -> (w385:cluster{dbl[], "Retract":dbl[]})  [unwired: 1 in]
        n181 = Bundle("PointsArray"=w373, "Approach"=w384) -> (w368:cluster{"PointsArray":dbl[], "Approach":dbl[]})  [unwired: 1 in]
        n182 = Bundle("PointsArray"=w373, "Approach"=w377) -> (w367:cluster{"PointsArray":dbl[], "Approach":dbl[]})  [unwired: 1 in]
        n183 = Bundle(w375, "Retract"=w376) -> (w374:cluster{dbl[], "Retract":dbl[]})  [unwired: 1 in]
        n184 = Build Array(w366, w385, w368, w378, w367, w374) -> (w365:cluster{"PointsArray":dbl[], "Retract":dbl[]}[])
      }
      frame "ForceCurve.AcquireBwd" {
      }
      frame "Graph.Update" {
        n185 = property on="ChannelDisplay2" class="Ring (strict)"() -> ("Value"=w468:u16)  [unwired: 2 in, 2 out]
        n186 = property on="ChannelDisplay" class="Ring (strict)"() -> ("Value"=w470:u16)  [unwired: 2 in, 2 out]
        n187 = Multiply(x=w470, y=u16 2) -> (x*y=w469:u16)
        n188 = property on="ChannelDisplay2" class="Ring (strict)"() -> ("Strings []"=w477:string[])  [unwired: 2 in, 2 out]
        n189 = property on="Bwd sweep" class="Bool (strict)" props=["Value"]() -> ()  [unwired: 2 in, 3 out]
        n190 = Increment(x=w469) -> (x+1=w473:u16)
        n191 = Index Array(array=w477, index=w468) -> (element=w461:string)
        n192 = property on="ChannelDisplay" class="Ring (strict)"() -> ("Strings []"=w466:string[])  [unwired: 2 in, 2 out]
        n193 = Multiply(x=w468, y=u16 2) -> (x*y=w467:u16)
        n194 = Increment(x=w467) -> (x+1=w471:u16)
        n195 = Index Array(array=w466, index=w470) -> (element=w463:string)
        n196 = Concatenate Strings(w461, " (V)" ("Y Scale.Unit Label.Text")) -> (w460:string)
        n197 = property on="ForceCurves 2" class="XYGraph (strict)"("YScale.NameLbl.Text"=w460) -> ()  [unwired: 2 in, 2 out]
        n198 = Concatenate Strings(w463, " (V)" ("Y Scale.Unit Label.Text")) -> (w462:string)
        n199 = property on="ForceCurves" class="XYGraph (strict)"("YScale.NameLbl.Text"=w462) -> ()  [unwired: 2 in, 2 out]
        n200 = Index Array(array=w475, index #1=w469, index #2=w473, index #3=w467, index #4=w471) -> (element #1=w483:cluster{"PointsArray":dbl[], "Retract":dbl[]}, element #2=w482:cluster{"PointsArray":dbl[], "Retract":dbl[]}, element #3=w480:cluster{"PointsArray":dbl[], "Retract":dbl[]}, element #4=w479:cluster{"PointsArray":dbl[], "Retract":dbl[]})
        n201 = Build Array(w483, w482) -> (→"ForceCurves":cluster{"PointsArray":dbl[], "Retract":dbl[]}[])
        n202 = Build Array(w480, w479) -> (→"ForceCurves 2":cluster{"PointsArray":dbl[], "Retract":dbl[]}[])
      }
      frame "Feedback.Reenable" {
        n203 = Multiply(x=0.05 ("y"), y=w489) -> (x*y=w491:dbl)
        n204 = Subtract(x=w489, y=w491) -> (x-y=w492:dbl)
        n205 = Increment(x=w492) -> (x+1=w509:dbl)
        n206 = xnode "Read/Write Control"("FPGA VI Reference In"=w498, "error in"=w497) -> ("FPGA VI Reference Out"=w496:T14, "error out"=w495:errorcluster, "fb.mot.p.params"=w494:T15)
        n207 = Bundle By Name(cluster=w494, "enableManualMotion"=TRUE, "doMove"=TRUE, "integratorTarget"=w509) -> (w493:T15)
        n208 = xnode "Read/Write Control"("FPGA VI Reference In"=w496, "error in"=w495, "fb.mot.p.params"=w493) -> ("FPGA VI Reference Out"=w488:T14, "error out"=w487:errorcluster)
        n209 = while {
          tunnel: w487 -> [w517]
          tunnel: w488 -> [w516]
          tunnel: [w515] -> w504
          tunnel: [w514] -> w508
          stop <- w513 stop-if-true
          n210 = xnode "Read/Write Control"("FPGA VI Reference In"=w516, "error in"=w517) -> ("FPGA VI Reference Out"=w515:T14, "error out"=w514:errorcluster, "fb.mot.s.running"=w512:bool)
          n211 = Not(x=w512) -> (.not. x?=w513:bool)
        }
        n212 = Bundle By Name(cluster=w493, "enableManualMotion"=FALSE, "doMove"=FALSE) -> (w503:T15)
        n213 = xnode "Read/Write Control"("FPGA VI Reference In"=w504, "error in"=w508, "fb.p.enable"=TRUE ("enableFeedback"), "fb.mot.p.params"=w503) -> ("FPGA VI Reference Out"=w499:T14, "error out"=w500:errorcluster)
      }
      frame "Save" {
        w526 = "\t"
        n214 = property on="Channels" class="LstBox (strict)"() -> ("Item Names"=w539:string[])  [unwired: 2 in, 2 out]
        n215 = Get Date/Time In Seconds() -> (seconds since 1Jan1904=w567:timestamp)
        n216 = Unbundle By Name("Saving") -> ("Path"=w553:path, "Name"=w568:string, "#"=w577:i64)
        n217 = local read "Channels"() -> (w534:i32[])
        n218 = Format Date/Time String(time format string (%c)="%H-%M-%S", seconds (now)=w567) -> (date/time string=w566:string)  [unwired: 1 in]
        n219 = for {
          tunnel: w539 -> [w592]
          tunnel: w534 -> [w593] mode=indexing
          shift-right: [w589] -> w528
          shift-left: "" -> [w591]
          w588 = "\t"
          n220 = Index Array(array=w592, index=w593) -> (element=w590:string)
          n221 = Concatenate Strings(w591, w590, w588, w588, w588) -> (w589:string)
        }
        n222 = property on="Parameters" class="Clust (strict)"() -> ("Controls[]"=w550:refnum<vi>[])  [unwired: 2 in, 2 out]
        n223 = Not Equal?(x=w568, y="") -> (x != y?=w544:bool)
        n224 = Concatenate Strings("Ramp_", w566) -> (w564:string)
        n225 = for {
          tunnel: w550 -> [w609] mode=indexing
          tunnel: [w604] -> w538 mode=indexing
          w601 = "\t"
          n226 = property class="Ctl"(reference=w609) -> ("Label.Text"=w605:string, "Value"=w608:variant)  [unwired: 1 in, 2 out]
          n227 = Variant To Data(type=0.0, Variant=w608) -> (data=w603:dbl)  [unwired: 1 in, 1 out]
          n228 = Format Value(format string="%.3e", value (0)=w603) -> (output string=w606:string)  [unwired: 1 in]
          n229 = Concatenate Strings(w605, w601, w606, w601) -> (w604:string)
        }
        n230 = Select(t=w568, s=w544, f=w564) -> (s? t:f=w541:string)
        n231 = Number To Decimal String(number=w577) -> (decimal integer string=w571:string)  [unwired: 1 in]
        n232 = Create Folder(path (use dialog)=w553) -> (created path=w552:path, error out=w549:errorcluster)  [unwired: 2 in, 1 out]
        n233 = Concatenate Strings(w541, "_" ("string"), w571) -> (w570:string)
        n234 = call <vilib>:"Clear Errors.vi"("error in (no error)"=w549, "specific error code to clear (0: all)"=10) -> ()  [unwired: 4 in, 2 out]
        n235 = Array Size(array=w534) -> (size(s)=w525:i32)
        n236 = Build Path(base path=w552, name or relative path=w570) -> (appended path=w562:path)
        n237 = Concatenate Strings("Forward (m)" ("string"), w526, w526, "Backward (m)" ("string"), w528, "\n") -> (w531:string)
        n238 = Multiply(x=w525, y=2 ("x")) -> (x*y=w530:i32)
        n239 = Open/Create/Replace File(file path (use dialog)=w562, error in=w574, operation (0:open)=T10."open or create") -> (refnum out=w551:refnum<file>, error out=w575:errorcluster)  [unwired: 3 in, 1 out]
        n240 = Equal?(x=FALSE, y=w544) -> (x = y?=w542:bool)
        n241 = Write to Text File "Header"(file (use dialog)=w551, text=w538, error in=w575) -> (refnum out=w536:refnum<file>, error out=w537:errorcluster)  [unwired: 1 in, 1 out]
        n242 = case shown="False" w542 {
          tunnel: w577 -> [w594 _]
          tunnel: [w594 i64 -1 ("#")] -> w543
          frame False {
          }
          frame True {
          }
        }
        n243 = for {
          N: w530 -> [_]
          tunnel: w518 -> [w587]
          shift-right: [w586] -> w522
          shift-left: dbl[][] [] -> [w584]
          i -> [w583]
          n244 = Quotient & Remainder(x=w583, y=2) -> (floor(x/y)=w581:i32)  [unwired: 1 out]
          n245 = Index Array(array=w587, index=w583) -> (element=w585:cluster{"PointsArray":dbl[], "Retract":dbl[]})
          n246 = Equal To 0?(x=w581) -> (x = 0?=w580:bool)
          n247 = Unbundle(w585) -> ("Retract"=w578:dbl[])  [unwired: 1 out]
          n248 = Select(t=w578, s=w580, f=w578) -> (s? t:f=w579:dbl[])
          n249 = Build Array (concatenate)(w584, w579) -> (w586:dbl[][])
        }
        n250 = Write to Text File "Names"(file (use dialog)=w536, text=w531, error in=w537) -> (refnum out=w535:refnum<file>, error out=w576:errorcluster)  [unwired: 1 in, 1 out]
        n251 = Index Array(array=w518) -> (element=w520:cluster{"PointsArray":dbl[], "Retract":dbl[]})  [unwired: 1 in]
        n252 = Unbundle(w520) -> ("PointsArray"=w519:dbl[])  [unwired: 1 out]
        n253 = Reverse 1D Array(array=w519) -> (reversed array=w523:dbl[])
        n254 = Build Array (concatenate)(w523, w519, w522) -> (w560:dbl[][])
        n255 = Transpose 2D Array(2D array=w560) -> (transposed array=w557:dbl[][])
        n256 = Array To Spreadsheet String(array=w557, 3:"%.9e" ("format string")) -> (spreadsheet string=w556:string)  [unwired: 1 in]
        n257 = Write to Text File "Data"(file (use dialog)=w535, text=w556, error in=w576) -> (refnum out=w559:refnum<file>, error out=w555:errorcluster)  [unwired: 1 in, 1 out]
        n258 = Close File(refnum=w559, error in=w555) -> (error out=w547:errorcluster)  [unwired: 1 out]
        n259 = case shown="No Error" w547 {
          tunnel: "Saving" -> [w600 _]
          tunnel: w543 -> [w598 _]
          frame No Error {
            n260 = Increment(x=w598) -> (x+1=w599:i64)
            n261 = Bundle By Name(cluster=w600, "#"=w599) -> (w597:T4)
            n262 = property on="Save" class="Bool (strict)"("Value"=FALSE) -> ()  [unwired: 2 in, 2 out]
            n263 = local write "Saving"(w597) -> ()
          }
          frame Error {
          }
        }
      }
      frame "SaveToImage" {
        w613 = TRUE ("Hide Grid")
        (unwired) 10 ("specific error code to clear (0: all)")
        n264 = local read "Saving"() -> (w614:T4)
        n265 = Variant To Data(error in=w643, type=refnum<vi> refnum ("CtlRef"), Variant=w641) -> (data=w639:refnum<vi>, error out=w637:errorcluster)
        n266 = Unbundle By Name(w614) -> ("Path"=w610:path, "Name"=w629:string, "#"=w624:i64)
        n267 = property class="Bool"(reference=w639, error in=w637) -> (error out=w648:errorcluster, "Owner"=w638:refnum<vi>)  [unwired: 1 out]
        n268 = Get Date/Time In Seconds() -> (seconds since 1Jan1904=w621:timestamp)
        n269 = Format Date/Time String(time format string (%c)="%H-%M-%S", seconds (now)=w621) -> (date/time string=w619:string)  [unwired: 1 in]
        n270 = Not Equal?(x=w629, y="") -> (x != y?=w625:bool)
        n271 = To More Specific Class(target class=refnum<vi> refnum ("Plot1"), reference=w638, error in=w648) -> (specific class reference=w635:refnum<vi>, error out=w634:errorcluster)
        n272 = Concatenate Strings("Ramp_", w619) -> (w627:string)
        n273 = Select(t=w629, s=w625, f=w627) -> (s? t:f=w623:string)
        n274 = Number To Decimal String(number=w624) -> (decimal integer string=w632:string)  [unwired: 1 in]
        n275 = property class="Clust"(reference=w635, error in=w634) -> (error out=w633:errorcluster, "Label.Text"=w612:string)  [unwired: 1 out]
        n276 = Create Folder(path (use dialog)=w610) -> (created path=w618:path, error out=w626:errorcluster)  [unwired: 2 in, 1 out]
        n277 = case shown="\"Plot1\"" w612 {
          tunnel: [w649 "" ("YScale.NameLbl.Text") w651] -> w611
          frame "Plot2" {
            n278 = property on="ForceCurves 2" class="XYGraph (strict)"() -> ("YScale.NameLbl.Text"=w649:string)  [unwired: 2 in, 2 out]
          }
          frame "Oops", Default {
          }
          frame "Plot1" {
            n279 = property on="ForceCurves" class="XYGraph (strict)"() -> ("YScale.NameLbl.Text"=w651:string)  [unwired: 2 in, 2 out]
          }
        }
        n280 = call <vilib>:"Clear Errors.vi"("error in (no error)"=w626) -> ()  [unwired: 5 in, 2 out]
        n281 = Concatenate Strings(w623, "_" ("string"), w632, w611) -> (w631:string)
        n282 = Build Path(base path=w618, name or relative path=w631) -> (appended path=w617:path)
        n283 = case shown="\"Plot1\"" w612 {
          tunnel: [w658 w659 w665] -> w642
          tunnel: w633 -> [w657 w659 _]
          tunnel: w617 -> [w656 _ w662]
          tunnel: enum32{"BMP", "EPS", "EMF", "PICT"}."BMP" ("File Type") -> [w655 _ w664]
          tunnel: enum32{"File", "Clipboard"}."File" ("Target") -> [w654 _ w663]
          tunnel: w613 -> [w653 _ w661]
          tunnel: w613 -> [w652 _ w660]
          frame "Plot2" {
            n284 = invoke on="ForceCurves 2" class="XYGraph (strict)" method="Export Image"(error in=w657, "FileType"=w655, "Target"=w654, "Path"=w656, "HideGrid"=w653, "Overwrite"=w652) -> (error out=w658:errorcluster)  [unwired: 2 in, 7 out]
          }
          frame Default {
          }
          frame "Plot1" {
            n285 = invoke on="ForceCurves" class="XYGraph (strict)" method="Export Image"("FileType"=w664, "Target"=w663, "Path"=w662, "HideGrid"=w661, "Overwrite"=w660) -> (error out=w665:errorcluster)  [unwired: 3 in, 7 out]
          }
        }
      }
      frame "Save.ChangeName" {
        n286 = property on="#" class="DigNum (strict)"(error in=w668, "Value"=i64 0) -> (error out=w667:errorcluster)  [unwired: 1 in, 1 out]
      }
      frame "Exit" {
        n287 = Release Queue(queue=w681, error in (no error)=w678) -> (error out=w679:errorcluster)  [unwired: 1 in, 2 out]
        n288 = Merge Errors(w679) -> (w677:errorcluster)
      }
      frame Default {
        n289 = Format Into String(format string="The message\"%s\" received in the gestion loop is not valid" ("Texte de message d'erreur inconnu"), w689) -> (resulting string=w686:string)  [unwired: 2 in, 1 out]
        n290 = call <vilib>:"Error Cluster From Error Code.vi"("error message (\"\")"=w686, "error code (0)"=1 ("code d'erreur (0)")) -> ("error out"=w687:errorcluster)  [unwired: 7 in]
      }
    }
  }
  n291 = disable-structure shown="Disabled" {
    frame Disabled {
      n292 = for {
        tunnel: _ -> [w706]
        tunnel: [w711] -> _
        tunnel: _ -> [w705]
        tunnel: [w712] -> _
        w700 = 7 ("IRQ Number(s)")
        n293 = xnode "Read/Write Control"("error in"=w706) -> ("error out"=w709:errorcluster, "fb.mot.p.params"=w708:T15)  [unwired: 1 in, 1 out]
        n294 = xnode "Invoke Method"("IRQ Number(s)"=w700) -> ("FPGA VI Reference Out"=w695:T14)  [unwired: 2 in, 1 out]
        n295 = Bundle By Name(cluster=w708, "moveDecimation"=w705) -> (w707:T15)  [unwired: 1 in]
        n296 = xnode "Read/Write Control"("FPGA VI Reference In"=w695) -> ("FPGA VI Reference Out"=w697:T14, "ort.p.waveSize"=w696:u16)  [unwired: 1 in, 1 out]
        n297 = xnode "Read/Write Control"("error in"=w709, "fb.mot.p.params"=w707) -> ("error out"=w704:errorcluster)  [unwired: 1 in, 1 out]
        n298 = for {
          N: w696 -> [_]
          tunnel: [w717] -> w693 mode=indexing
          tunnel: w697 -> [w715]
          tunnel: [w714] -> w711
          tunnel: [w713] -> w712
          i -> [w716]
          n299 = xnode "Read/Write Control"("FPGA VI Reference In"=w715, "lwr.p.readAddress"=w716) -> ("FPGA VI Reference Out"=w719:T14, "error out"=w718:errorcluster)  [unwired: 1 in]
          n300 = xnode "Read/Write Control"("FPGA VI Reference In"=w719, "error in"=w718) -> ("FPGA VI Reference Out"=w713:T14, "error out"=w714:errorcluster, "lwr.o.readData"=w717:i32)
        }
        n301 = while {
          tunnel: w704 -> [w724]
          tunnel: [w721] -> w703
          tunnel: [w720] -> w702
          stop <- w722 continue-if-true
          n302 = xnode "Read/Write Control"("error in"=w724) -> ("FPGA VI Reference Out"=w721:T14, "error out"=w720:errorcluster, "fb.mot.s.running"=w722:bool)  [unwired: 1 in]
          n303 = Wait (ms)(milliseconds to wait=u32 10) -> ()  [unwired: 1 out]
        }
        n304 = xnode "Read/Write Control"("FPGA VI Reference In"=w703, "error in"=w702, "lwr.p.start"=TRUE) -> ("FPGA VI Reference Out"=w698:T14, "error out"=w710:errorcluster)
        n305 = property on="Sweeps" class="DigNum (strict)"() -> ("Value"=w692:dbl)  [unwired: 2 in, 2 out]
        n306 = To Word Integer(number=w692) -> (16bit integer=w691:i16)
        n307 = Negate(x=w691) -> ()  [unwired: 1 out]
        n308 = xnode "Invoke Method"("FPGA VI Reference In"=w698, "error in"=w710, "IRQ Number(s)"=w700, "Timeout (ms)"=1000) -> ()  [unwired: 4 out]
        n309 = To Double Precision Float(number=w693) -> (double precision float=w694:dbl[])
        n310 = Scale By Power Of 2(n=w691, x=w694) -> ()  [unwired: 1 out]
      }
    }
    frame Enabled {
    }
  }
  n311 = Merge Errors(w2, w6) -> (w8:errorcluster)
  n312 = disable-structure shown="Disabled" {
    disable-tunnel: w8 -> [w727 w728]
    disable-tunnel: [w726 w728] -> w7
    disable-tunnel: w5 -> [w725 _]
    frame Disabled {
      n313 = xnode "Close FPGA VI Reference"("FPGA VI Reference In"=w725, "error in"=w727) -> ("error out"=w726:errorcluster)
    }
    frame Enabled {
    }
  }
  n314 = call <vilib>:"Simple Error Handler.vi"("error in (no error)"=w7) -> ()  [unwired: 4 in, 5 out]
